vi "Xi^2-Xi-1^2.vi"(10 "X[-1]":dbl, 11 "Xi":dbl[](array[numeric])) -> (3 "Yi":dbl[](array[numeric]) format="%.2f")   [LabVIEW 2011]
doc: "Calculate sums of consecutive array elements. 0th element of output is equal to x(0)+ x(-1), where x(-1) is an optional scalar input that defaults to zero."
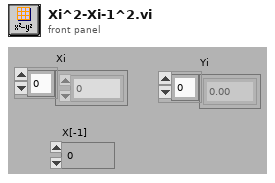
[diagram p1: front panel]
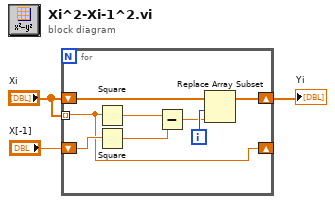
[diagram p0: block diagram]
diagram:
  n1 = for {
    shift-right: [w10] -> w1
    shift-left: "Xi" -> [w11]
    shift-right: [w4] -> _
    shift-left: "X[-1]" -> [w8]
    tunnel: "Xi" -> [w4] mode=indexing
    i -> [w9]
    n2 = Square(x=w4) -> (x^2=w6:dbl)
    n3 = Square(x=w8) -> (x^2=w5:dbl)
    n4 = Subtract(x=w6, y=w5) -> (x-y=w7:dbl)
    n5 = Replace Array Subset(array=w11, new element=w7, index=w9) -> (w10:dbl[])
  }
  "Yi" <- w1
